vi "rsp_Server Port Open.vi"(8 "error in":errorcluster, 9 "Placeholder":T1, 11 "DS TCP Server in":refnum<class "DS TCP Server.lvclass">) -> (0 "error out":errorcluster, 3 "dup DS TCP Server out":refnum<class "DS TCP Server.lvclass">)   [LabVIEW 2017, in "DS TCP Server.lvlib" / "DS TCP Server.lvclass"]
doc: "This VI sends a <b>Public API Response</b> message to a registered MHL case of the Caller of the Worker that owns this VI.\n---"
uses:
  DS TCP Server.lvclass
  C:/Program Files (x86)/National Instruments/LabVIEW 2017/vi.lib/addons/_Workers/Library/Classes/Worker/Worker.lvclass
  rsp_Server Port Open.ctl
  DS TCP Server.lvclass/DS TCP Server.ctl
  <vilib>/addons/_Workers/Library/Classes/Worker/Worker.lvclass/Worker.ctl
  <vilib>/addons/_Workers/Library/Classes/Message/Priority.ctl
  <vilib>/Utility/error.llb/Error Cluster From Error Code.vi
  <vilib>/addons/_Workers/Library/Classes/Message/Enqueue Message to Queue.vi
  <vilib>/ErrorRing/Error Ring.xnode
  <vilib>/addons/_Workers/Library/Classes/Message/Message.lvclass
  <vilib>/addons/_Workers/Library/Classes/Worker/Worker.lvclass
  C:/Program Files (x86)/National Instruments/LabVIEW 2017/vi.lib/addons/_Workers/Library/Classes/Workers Object/Workers Object.lvclass
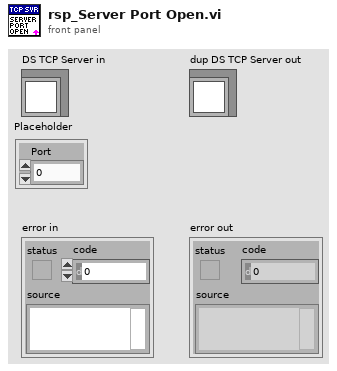
[diagram p1: front panel]
types:
  T1 = typedef "DS TCP Server.lvlib/DS TCP Server.lvclass/rsp_Server Port Open.ctl" = cluster{"Port":u16}
  T2 = typedef "Workers.lvlib/Case Label.ctl" = string
  T3 = typedef "Workers.lvlib/Message.lvclass/Priority.ctl" = enum16{"Low", "Normal", "High"}
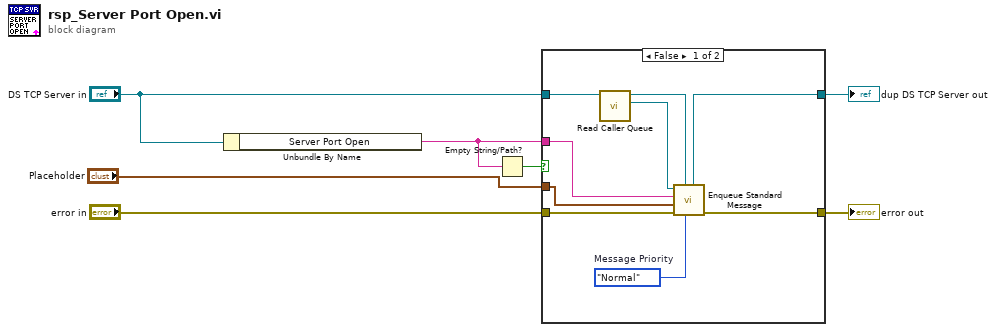
[diagram p0: block diagram]
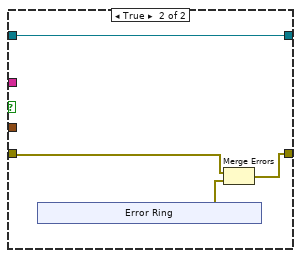
[diagram p2: hidden frame]
diagram:
  n1 = Unbundle By Name("DS TCP Server in") -> ("Server Port Open"=w3:T2)
  n2 = Empty String/Path?(string/path=w3) -> (empty?=w4:bool)
  n3 = case shown="False" w4 {
    tunnel: "error in" -> [w11 w18]
    tunnel: [w16 w17] -> w6
    tunnel: [w14 w20] -> w5
    tunnel: "DS TCP Server in" -> [w12 w20]
    tunnel: w3 -> [w13 _]
    tunnel: "Placeholder" -> [w8 _]
    frame False {
      w15 = Priority."Normal"  # Message Priority
      n4 = call <vilib>:"Read Caller Queue.vi"("Worker_"=w12) -> ("Message Queue out"=w9:refnum<class "Message Queue.lvclass">, "dup Worker_out"=w10:refnum<class "DS TCP Server.lvclass">)  [unwired: 9 in]
      n5 = call-poly <vilib>:"Enqueue Standard Message.vi"("Priority (Normal)"=w15, "Worker"=w10, "error in"=w11, "Data"=w8, "Case Label"=w13, "Message Queue"=w9) -> ("error out"=w16:errorcluster, "dup Worker out"=w14:refnum<class "DS TCP Server.lvclass">)  [unwired: 3 in, 1 out]
    }
    frame True {
      n6 = xnode "Error Ring"() -> ("error out"=w19:errorcluster)
      n7 = Merge Errors(w18, w19) -> (w17:errorcluster)
    }
  }
  "error out" <- w6
  "dup DS TCP Server out" <- w5
